vi "popUPInsertarTuplaEnDBReceta.vi"() -> (3 "Listo Ingresar OD SteelGrade Lote":bool=TRUE)   [LabVIEW 2014]
panel:
  in  "textoFinCarga":string="Gracias por ingresar los datos del producto"
  in  "guardarEnDBObjetoReceta":bool
  in  "idStadistic":string="idStadistic"
  in  "dataCreate":string="dateCreate"
  in  "idRecipe":string="idRecipe"
  in  "camposMedicion":string="numLote"
  in  "ingresarSteelGrade":string="numSteelGrade"
  in  "ingresarOD":string="numeroOD"
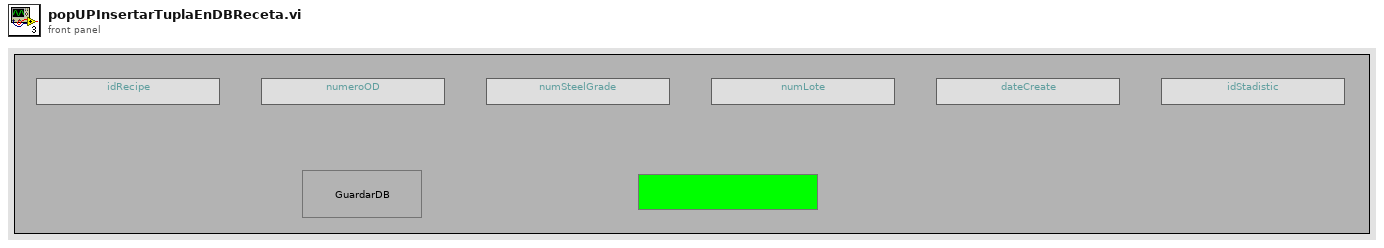
[diagram p1: front panel]
types:
  T1 = enum8{"Enabled", "Disabled", "Disabled and Grayed Out"}
  T2 = cluster{"idRecipe":string, "od":string, "sg":string, "camposMedicion":string, "dateCreate":string, "idStadistic":string}
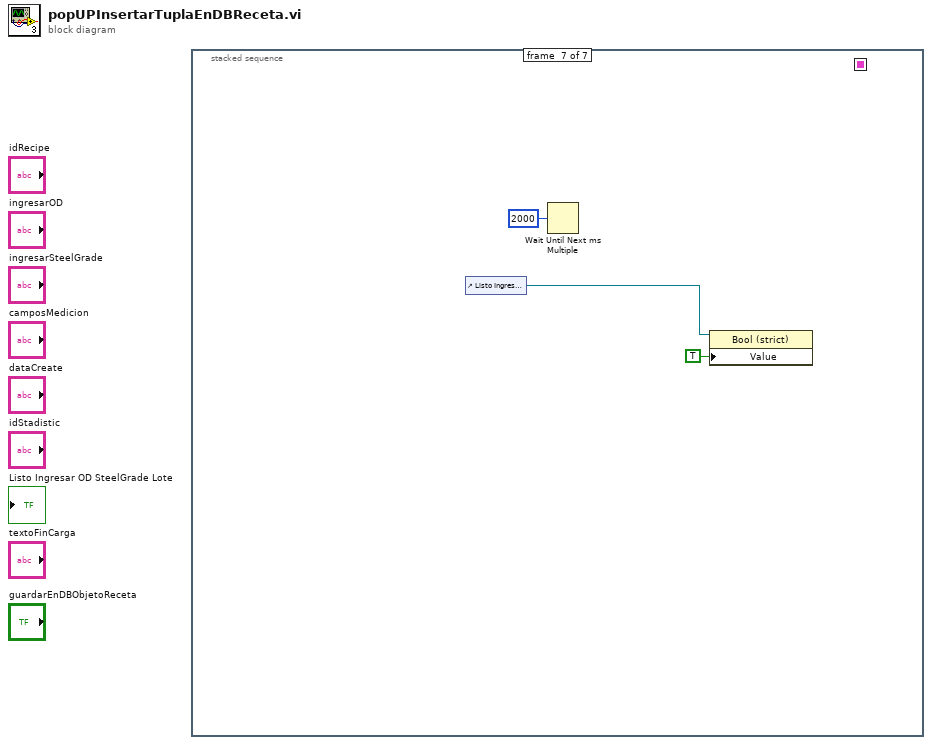
[diagram p0: block diagram]
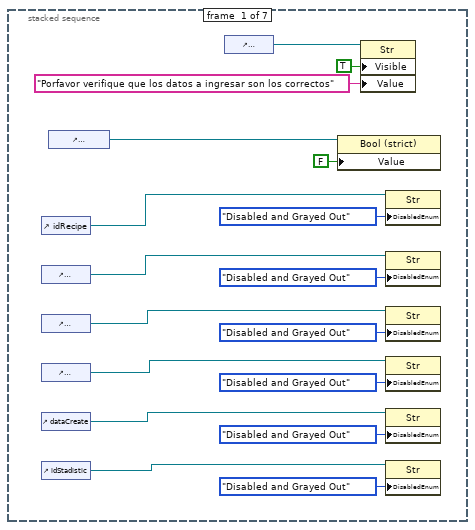
[diagram p2: hidden frame]
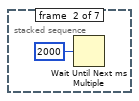
[diagram p3: hidden frame]
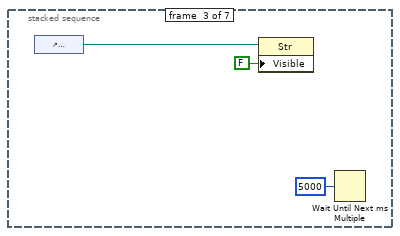
[diagram p4: hidden frame]
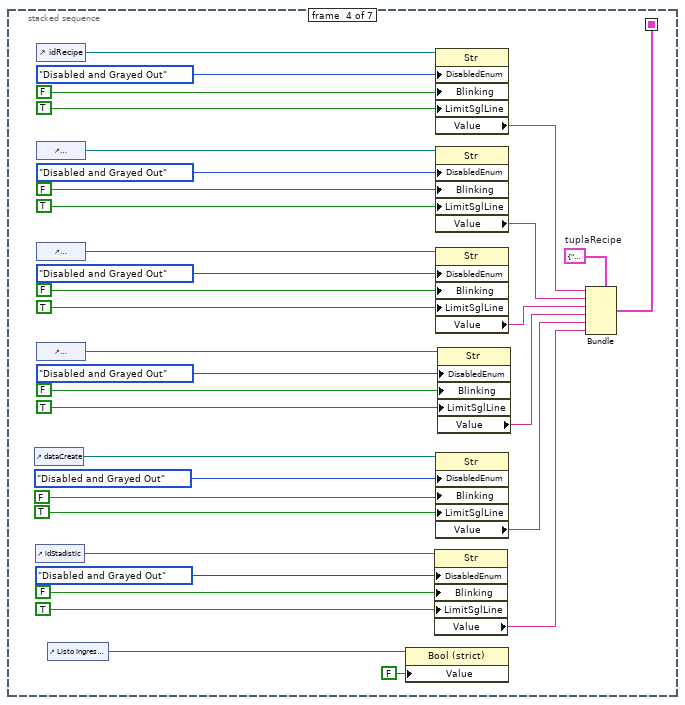
[diagram p5: hidden frame]
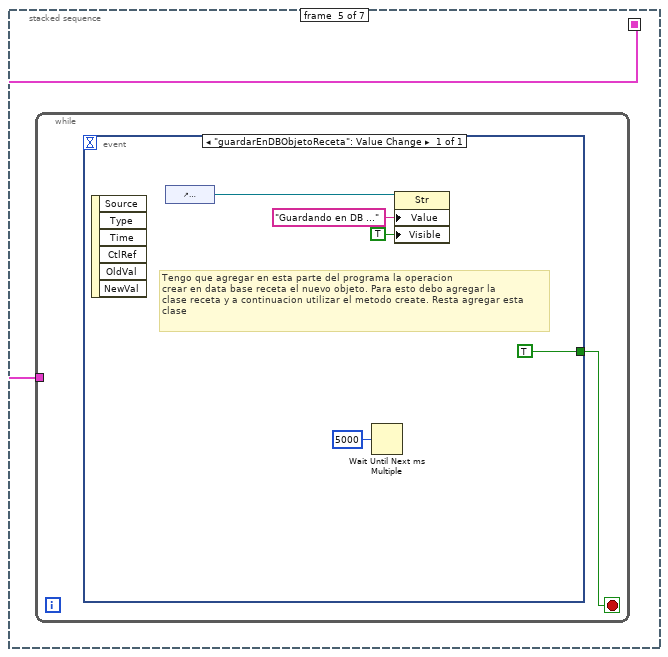
[diagram p6: hidden frame]
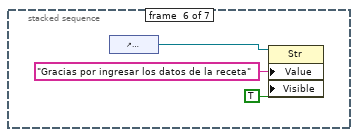
[diagram p7: hidden frame]
diagram:
  n1 = stacked-sequence {
    seq-local: [_ _ _ w22 _ _ _] -> [_ _ _ _ w56 _ _]
    frame #0 {
      n2 = control-ref of="idRecipe"() -> (w12:refnum<vi>)
      n3 = control-ref of="ingresarOD"() -> (w11:refnum<vi>)
      n4 = control-ref of="ingresarSteelGrade"() -> (w10:refnum<vi>)
      n5 = control-ref of="camposMedicion"() -> (w9:refnum<vi>)
      n6 = control-ref of="dataCreate"() -> (w8:refnum<vi>)
      n7 = control-ref of="idStadistic"() -> (w7:refnum<vi>)
      n8 = control-ref of="guardarEnDBObjetoReceta"() -> (w14:refnum<vi>)
      n9 = control-ref of="textoFinCarga"() -> (w17:refnum<vi>)
      n10 = property class="Bool (strict)"(reference=w14, "Value"=FALSE) -> ()  [unwired: 1 in, 2 out]
      n11 = property class="Str"(reference=w17, "Visible"=TRUE, "Value"="Porfavor verifique que los datos a ingresar son los correctos") -> ()  [unwired: 1 in, 2 out]
      n12 = property class="Str"(reference=w12, "DisabledEnum"=T1."Disabled and Grayed Out" ("Disabled")) -> ()  [unwired: 1 in, 2 out]
      n13 = property class="Str"(reference=w11, "DisabledEnum"=T1."Disabled and Grayed Out" ("Disabled")) -> ()  [unwired: 1 in, 2 out]
      n14 = property class="Str"(reference=w10, "DisabledEnum"=T1."Disabled and Grayed Out" ("Disabled")) -> ()  [unwired: 1 in, 2 out]
      n15 = property class="Str"(reference=w9, "DisabledEnum"=T1."Disabled and Grayed Out" ("Disabled")) -> ()  [unwired: 1 in, 2 out]
      n16 = property class="Str"(reference=w8, "DisabledEnum"=T1."Disabled and Grayed Out" ("Disabled")) -> ()  [unwired: 1 in, 2 out]
      n17 = property class="Str"(reference=w7, "DisabledEnum"=T1."Disabled and Grayed Out" ("Disabled")) -> ()  [unwired: 1 in, 2 out]
    }
    frame #1 {
      n18 = Wait Until Next ms Multiple(millisecond multiple=u32 2000) -> ()  [unwired: 1 out]
    }
    frame #2 {
      n19 = control-ref of="textoFinCarga"() -> (w21:refnum<vi>)
      n20 = property class="Str"(reference=w21, "Visible"=FALSE) -> ()  [unwired: 1 in, 2 out]
      n21 = Wait Until Next ms Multiple(millisecond multiple=u32 5000) -> ()  [unwired: 1 out]
    }
    frame #3 {
      w23 = T2 {"idRecipe"="", "od"="", "sg"="", "camposMedicion"="", "dateCreate"="", "idStadistic"=""}  # tuplaRecipe
      n22 = control-ref of="dataCreate"() -> (w37:refnum<vi>)
      n23 = control-ref of="idStadistic"() -> (w33:refnum<vi>)
      n24 = control-ref of="idRecipe"() -> (w41:refnum<vi>)
      n25 = control-ref of="ingresarOD"() -> (w55:refnum<vi>)
      n26 = control-ref of="ingresarSteelGrade"() -> (w53:refnum<vi>)
      n27 = control-ref of="camposMedicion"() -> (w51:refnum<vi>)
      n28 = control-ref of="Listo Ingresar OD SteelGrade Lote"() -> (w43:refnum<vi>)
      n29 = property class="Bool (strict)"(reference=w43, "Value"=FALSE) -> ()  [unwired: 1 in, 2 out]
      n30 = property class="Str"(reference=w33, "DisabledEnum"=T1."Disabled and Grayed Out" ("Disabled"), "Blinking"=FALSE, "LimitSglLine"=TRUE ("Limit To Single Line?")) -> ("Value"=w24:string)  [unwired: 1 in, 2 out]
      n31 = property class="Str"(reference=w41, "DisabledEnum"=T1."Disabled and Grayed Out" ("Disabled"), "Blinking"=FALSE, "LimitSglLine"=TRUE ("Limit To Single Line?")) -> ("Value"=w29:string)  [unwired: 1 in, 2 out]
      n32 = property class="Str"(reference=w55, "DisabledEnum"=T1."Disabled and Grayed Out" ("Disabled"), "Blinking"=FALSE, "LimitSglLine"=TRUE ("Limit To Single Line?")) -> ("Value"=w28:string)  [unwired: 1 in, 2 out]
      n33 = property class="Str"(reference=w53, "DisabledEnum"=T1."Disabled and Grayed Out" ("Disabled"), "Blinking"=FALSE, "LimitSglLine"=TRUE ("Limit To Single Line?")) -> ("Value"=w27:string)  [unwired: 1 in, 2 out]
      n34 = property class="Str"(reference=w37, "DisabledEnum"=T1."Disabled and Grayed Out" ("Disabled"), "Blinking"=FALSE, "LimitSglLine"=TRUE ("Limit To Single Line?")) -> ("Value"=w25:string)  [unwired: 1 in, 2 out]
      n35 = property class="Str"(reference=w51, "DisabledEnum"=T1."Disabled and Grayed Out" ("Disabled"), "Blinking"=FALSE, "LimitSglLine"=TRUE ("Limit To Single Line?")) -> ("Value"=w26:string)  [unwired: 1 in, 2 out]
      n36 = Bundle(cluster=w23, "idRecipe"=w29, "od"=w28, "sg"=w27, "camposMedicion"=w26, "dateCreate"=w25, "idStadistic"=w24) -> (w22:T2)
    }
    frame #4 {
      n37 = while {
        tunnel: w56 -> [_]
        stop <- w57 stop-if-true
        n38 = event shown="[0] \"guardarEnDBObjetoReceta\": Value Change" {
          selector: _ -> [_]
          dyn-events: _ -> [_]
          timeout: _ -> [_]
          tunnel: [TRUE] -> w57
          event "guardarEnDBObjetoReceta": Value Change {
            # "Tengo que agregar en esta parte del programa la operacion\ncrear en data base receta el nuevo objeto. Para esto debo agregar la \nclase receta y a continuacion utilizar el metodo create. Resta agregar esta \nclase"
            n39 = event-data() -> ()  [unwired: 1 in, 6 out]
            n40 = control-ref of="textoFinCarga"() -> (w62:refnum<vi>)
            n41 = Wait Until Next ms Multiple(millisecond multiple=u32 5000) -> ()  [unwired: 1 out]
            n42 = property class="Str"(reference=w62, "Value"="Guardando en DB ...", "Visible"=TRUE) -> ()  [unwired: 1 in, 2 out]
          }
        }
      }
    }
    frame #5 {
      n43 = control-ref of="textoFinCarga"() -> (w65:refnum<vi>)
      n44 = property class="Str"(reference=w65, "Value"="Gracias por ingresar los datos de la receta", "Visible"=TRUE) -> ()  [unwired: 1 in, 2 out]
    }
    frame #6 {
      n45 = control-ref of="Listo Ingresar OD SteelGrade Lote"() -> (w67:refnum<vi>)
      n46 = Wait Until Next ms Multiple(millisecond multiple=u32 2000) -> ()  [unwired: 1 out]
      n47 = property class="Bool (strict)"(reference=w67, "Value"=TRUE) -> ()  [unwired: 1 in, 2 out]
    }
  }
